vi "Move.vi"(4 "Units (0: microsteps)":u16(ring) items=["microsteps", "microns", "millimeters", "inches", "degrees"], 6 "Movement Type (0: relative)":u16(ring) items=["relative", "absolute"], 7 "Move Distance (0)":dbl, 8 "error in (no error)":errorcluster, 9 "Device and Axis":string, 10 "Microstep Size (0)":dbl, 11 "VISA resource name":refnum<visa-resource-name>) -> (0 "error out":errorcluster, 3 "VISA resource name out":refnum<visa-resource-name>)   [LabVIEW 2021, in "Zaber A Series.lvlib"]
doc: "Moves a device. You can optionally input the Device and Axis to move, and the other inputs specify the type of movement (absolute or relative), the units of the data you would like to send, and the distance data in those units. If no movement type or unit is input the default is relative movement in microsteps. Finally if you are using any other unit than microsteps you must input the Microstep Size for the model. \n\nNo responses are returned with this VI, but if you would like to wait until the movement is completed to continue, you can combine this VI with the Poll Until Idle VI. \n\nThis VI requires that the Initialize VI has been called with the same serial port. \n\nNote: See the Device Lookup control for the microstep size of your model, or check on the product specifications page for the product on www.zaber.com."
uses:
  Zaber A Series.lvlib
  Private/Basic Commands.ctl
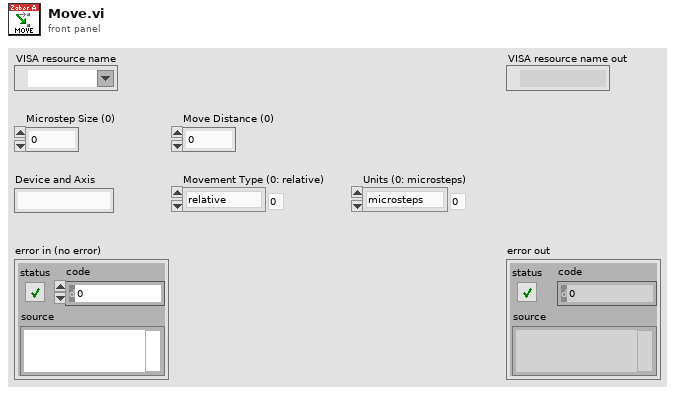
[diagram p1: front panel]
types:
  T1 = typedef "Zaber A Series.lvlib/Basic Commands.ctl" = string
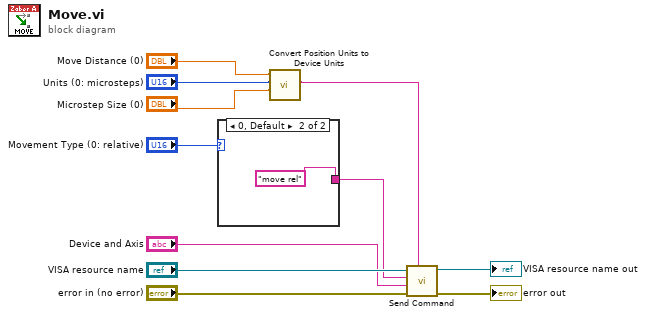
[diagram p0: block diagram]
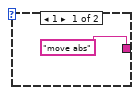
[diagram p2: hidden frame]
diagram:
  n1 = case shown="0, Default" "Movement Type (0: relative)" {
    tunnel: [T1 "move abs" ("Basic Command List") T1 "move rel" ("Basic Command List")] -> w9
    frame 1 {
    }
    frame 0, Default {
    }
  }
  n2 = call "Convert Position Units to Device Units.vi"("Microstep Size (0)"="Microstep Size (0)", "Units (0: microsteps)"="Units (0: microsteps)", "Position (0)"="Move Distance (0)") -> ("Device Position (String)"=w6:string)  [unwired: 6 in, 2 out]
  n3 = call "Send Command.vi"("Data"=w6, "error in (no error)"="error in (no error)", "Device and Axis"="Device and Axis", "Command"=w9, "VISA resource name"="VISA resource name") -> ("error out"=→"error out":errorcluster, "VISA resource name out"=→"VISA resource name out":refnum<visa-resource-name>)  [unwired: 1 in, 4 out]
